vi "WriteIOSafeCondition b2g1.vi"(1 "error in":errorcluster) -> (0 "error out":errorcluster)   [LabVIEW 2011]
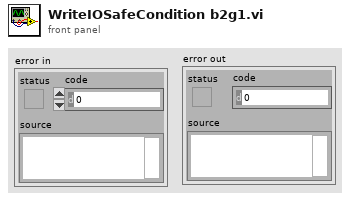
[diagram p1: front panel]
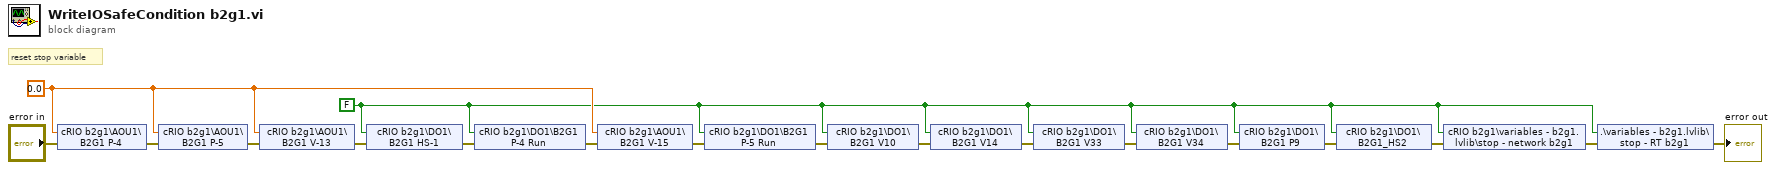
[diagram p0: block diagram]
diagram:
  w3 = FALSE ("B2G1 P-4")
  w10 = 0.0 ("B2G1 V-13")
  # "reset stop variable"
  n1 = shared-variable "cRIO b2g1\\AOU1\\B2G1 P-4"(w10, error in="error in") -> (error out=w14:errorcluster)
  n2 = shared-variable "cRIO b2g1\\AOU1\\B2G1 P-5"(w10, error in=w14) -> (error out=w18:errorcluster)
  n3 = shared-variable "cRIO b2g1\\AOU1\\B2G1 V-13"(w10, error in=w18) -> (error out=w17:errorcluster)
  n4 = shared-variable "cRIO b2g1\\DO1\\B2G1 HS-1"(w3, error in=w17) -> (error out=w13:errorcluster)
  n5 = shared-variable "cRIO b2g1\\DO1\\B2G1 P-4 Run"(w3, error in=w13) -> (error out=w15:errorcluster)
  n6 = shared-variable "cRIO b2g1\\AOU1\\B2G1 V-15"(w10, error in=w15) -> (error out=w8:errorcluster)
  n7 = shared-variable "cRIO b2g1\\DO1\\B2G1 P-5 Run"(w3, error in=w8) -> (error out=w7:errorcluster)
  n8 = shared-variable "cRIO b2g1\\DO1\\B2G1 V10"(w3, error in=w7) -> (error out=w12:errorcluster)
  n9 = shared-variable "cRIO b2g1\\DO1\\B2G1 V14"(w3, error in=w12) -> (error out=w16:errorcluster)
  n10 = shared-variable "cRIO b2g1\\DO1\\B2G1 V33"(w3, error in=w16) -> (error out=w9:errorcluster)
  n11 = shared-variable "cRIO b2g1\\DO1\\B2G1 V34"(w3, error in=w9) -> (error out=w4:errorcluster)
  n12 = shared-variable "cRIO b2g1\\DO1\\B2G1 P9"(w3, error in=w4) -> (error out=w2:errorcluster)
  n13 = shared-variable "cRIO b2g1\\DO1\\B2G1_HS2"(w3, error in=w2) -> (error out=w1:errorcluster)
  n14 = shared-variable "cRIO b2g1\\variables - b2g1.lvlib\\stop - network b2g1"(w3, error in=w1) -> (error out=w11:errorcluster)
  n15 = shared-variable ".\\variables - b2g1.lvlib\\stop - RT b2g1"(w3, error in=w11) -> (error out=→"error out":errorcluster)
